vi "Write Captions.vi"(8 "error in (no error)":errorcluster, 10 "Captions and counters":T8, 11 "PDF Report Class in":refnum<class "PDF Report Class.lvclass">) -> (0 "error out":errorcluster, 3 "PDF Report Class out":refnum<class "PDF Report Class.lvclass">)   [LabVIEW 2019, in "Exaprom PDF.lvlib" / "PDF Report Class.lvclass"]
uses:
  PDF Report Class.lvclass
  Controls/Initialization Controls/Captions.ctl
  Controls/Initialization Controls/Image or Table Caption.ctl
  Controls/Font Controls/Font complete cluster.ctl
  Controls/Font Controls/Font size.ctl
  Controls/Font Controls/Font color.ctl
  Controls/Font Controls/Type and encoding.ctl
  Controls/Text Controls/Unicode/Type and run direction.ctl
  PDF Report Class.lvclass/PDF Report Class.ctl
  Exaprom PDF.lvlib
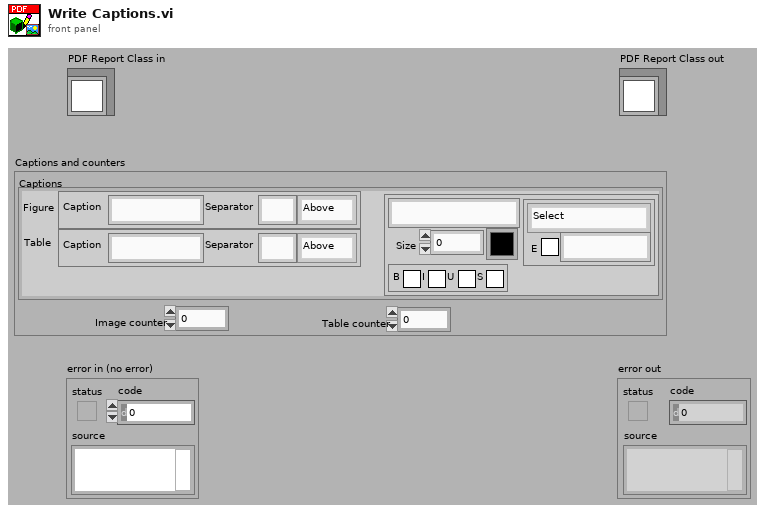
[diagram p1: front panel]
types:
  T1 = typedef "Exaprom PDF.lvlib/Captions.ctl" = cluster{"Figure":T2, "Table":T2, "Font":T3}
  T2 = typedef "Exaprom PDF.lvlib/Image or Table Caption.ctl" = cluster{"Caption":string, "Separator":string, "Position":enum16{"Above", "Below"}}
  T3 = typedef "Exaprom PDF.lvlib/Font complete cluster.ctl" = cluster{"Name":string, "Size":T4, "Color":T5, "Style":cluster{"Bold":bool, "Italic":bool, "Underline":bool, "Strikeout":bool}, "Type":T6}
  T4 = typedef "Exaprom PDF.lvlib/Font size.ctl" = sgl
  T5 = typedef "Exaprom PDF.lvlib/Font color.ctl" = u32
  T6 = typedef "Exaprom PDF.lvlib/Type and encoding.ctl" = cluster{"Type&direction":T7, "Embedded":bool, "Encoding":string}
  T7 = typedef "Exaprom PDF.lvlib/Type and run direction.ctl" = enum16{"Select", "ASCII", "UTF-16", "UTF-16 (default)", "UTF-16 (LTR)", "UTF-16 (RTL)"}
  T8 = cluster{"Captions":T1, "Image counter":u16, "Table counter":u16}
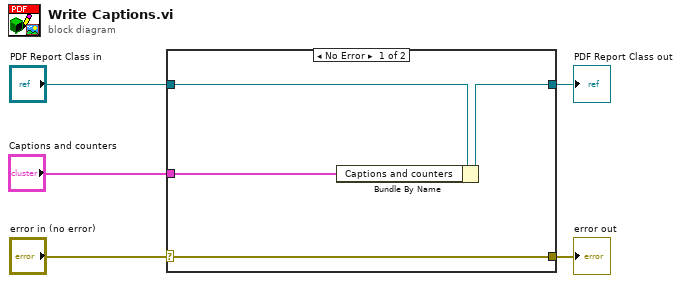
[diagram p0: block diagram]
diagram:
  n1 = case shown="No Error" "error in (no error)" {
    selector: "error in (no error)" -> [w9 w10]
    tunnel: [w9 w10] -> w4
    tunnel: [w7 w11] -> w2
    tunnel: "PDF Report Class in" -> [w8 w11]
    tunnel: "Captions and counters" -> [w6 _]
    frame No Error {
      n2 = Bundle By Name(cluster=w8, "Captions and counters"=w6) -> (w7:refnum<class "PDF Report Class.lvclass">)
    }
    frame Error {
    }
  }
  "error out" <- w4
  "PDF Report Class out" <- w2
